vi "SW Arch main.vi"() -> ()   [LabVIEW 2009]
uses:
  <vilib>/Platform/TimedLoop/XDataNode/XDataNode.xnode
  <vilib>/Platform/TimedLoop/XDataNode/nitl_modes.ctl
  <vilib>/Platform/TimedLoop/XDataNode/XDNodeRunTimeDep.lvlib
  <vilib>/Platform/TimedLoop/XDataNode/wakeup.ctl
  <vilib>/Platform/TimedLoop/XDataNode/timing_clust.ctl
  <vilib>/Platform/TimedLoop/XDataNode/loadlvalarms.vi
  <vilib>/rvi/interface/nirviOpenFPGA/nirviOpenFPGA.xnode
  <vilib>/userDefined/High Color/nirio_resource_hc.ctl
  Remote Control/Motor Command.ctl
  TypeDefs/Queue TypeDefs/Motor Instruction.ctl
  TypeDefs/State Machine/Main State.ctl
  <vilib>/LabVIEW Targets/FPGA/cRIO/shared/nicrio_ModuleControls/nicrio_cRIO-9871_DataBitsEnum.ctl
  <vilib>/LabVIEW Targets/FPGA/cRIO/shared/nicrio_ModuleControls/nicrio_cRIO-9871_FlowControlEnum.ctl
  <vilib>/LabVIEW Targets/FPGA/cRIO/shared/nicrio_ModuleControls/nicrio_cRIO-9871_BaudRateEnum.ctl
  <vilib>/LabVIEW Targets/FPGA/cRIO/shared/nicrio_ModuleControls/nicrio_cRIO-9871_ParityEnum.ctl
  <vilib>/LabVIEW Targets/FPGA/cRIO/shared/nicrio_ModuleControls/nicrio_cRIO-9871_StopBitsEnum.ctl
  Remote Control/Message Type.ctl
  FPGA Bitfiles/Q_IGVC_2010.lvproj_FPGA Target_FPGA_MAIN.vi.lvbitx
  TypeDefs/Queue TypeDefs/Motor State.ctl
  <vilib>/FPGAPlugInAG/cRIO-9113/nirviIntfOpen_cRIO-9113.vi
  TypeDefs/Sensor TypeDefs/FPGA Main ref.ctl
  TypeDefs/Sensor TypeDefs/GPS Data.ctl
  TypeDefs/Sensor TypeDefs/SICK Array.ctl
  Remote Control/Control Message.ctl
panel:
  in  "Control Message":T1
  in  "Read Timeout":i32=1000
  in  "Local Port":u16=8800
  out "Run/!RC":bool=TRUE
  out "Main State":T3=enum."Initialize Sensors"
  out "MC VISA resource":refnum<visa-resource-name>="ASRL1::INSTR"
  in  "Motors Init Complete":bool
  out "Motor Queue":refnum<queue>
  in  "RC Command Buffer":T2
  in  "Motors On?":bool
  in  "Sensors Init Complete":bool
  in  "SICK Buffer":T4
  in  "Compass Buffer":dbl=181.1
  in  "Compass Init Complete":bool
  in  "SICK Init Complete":bool
  in  "GPS Init Complete":bool
  in  "GPS Buffer":T5 {"Longitude" format="%#_14g"; "Latitude" format="%#_14g"}
  out "FPGA VI Reference":T6
  in  "Motor Message":string
  out "VFH Queue":refnum<queue>
  out "Communication Queue":refnum<queue>
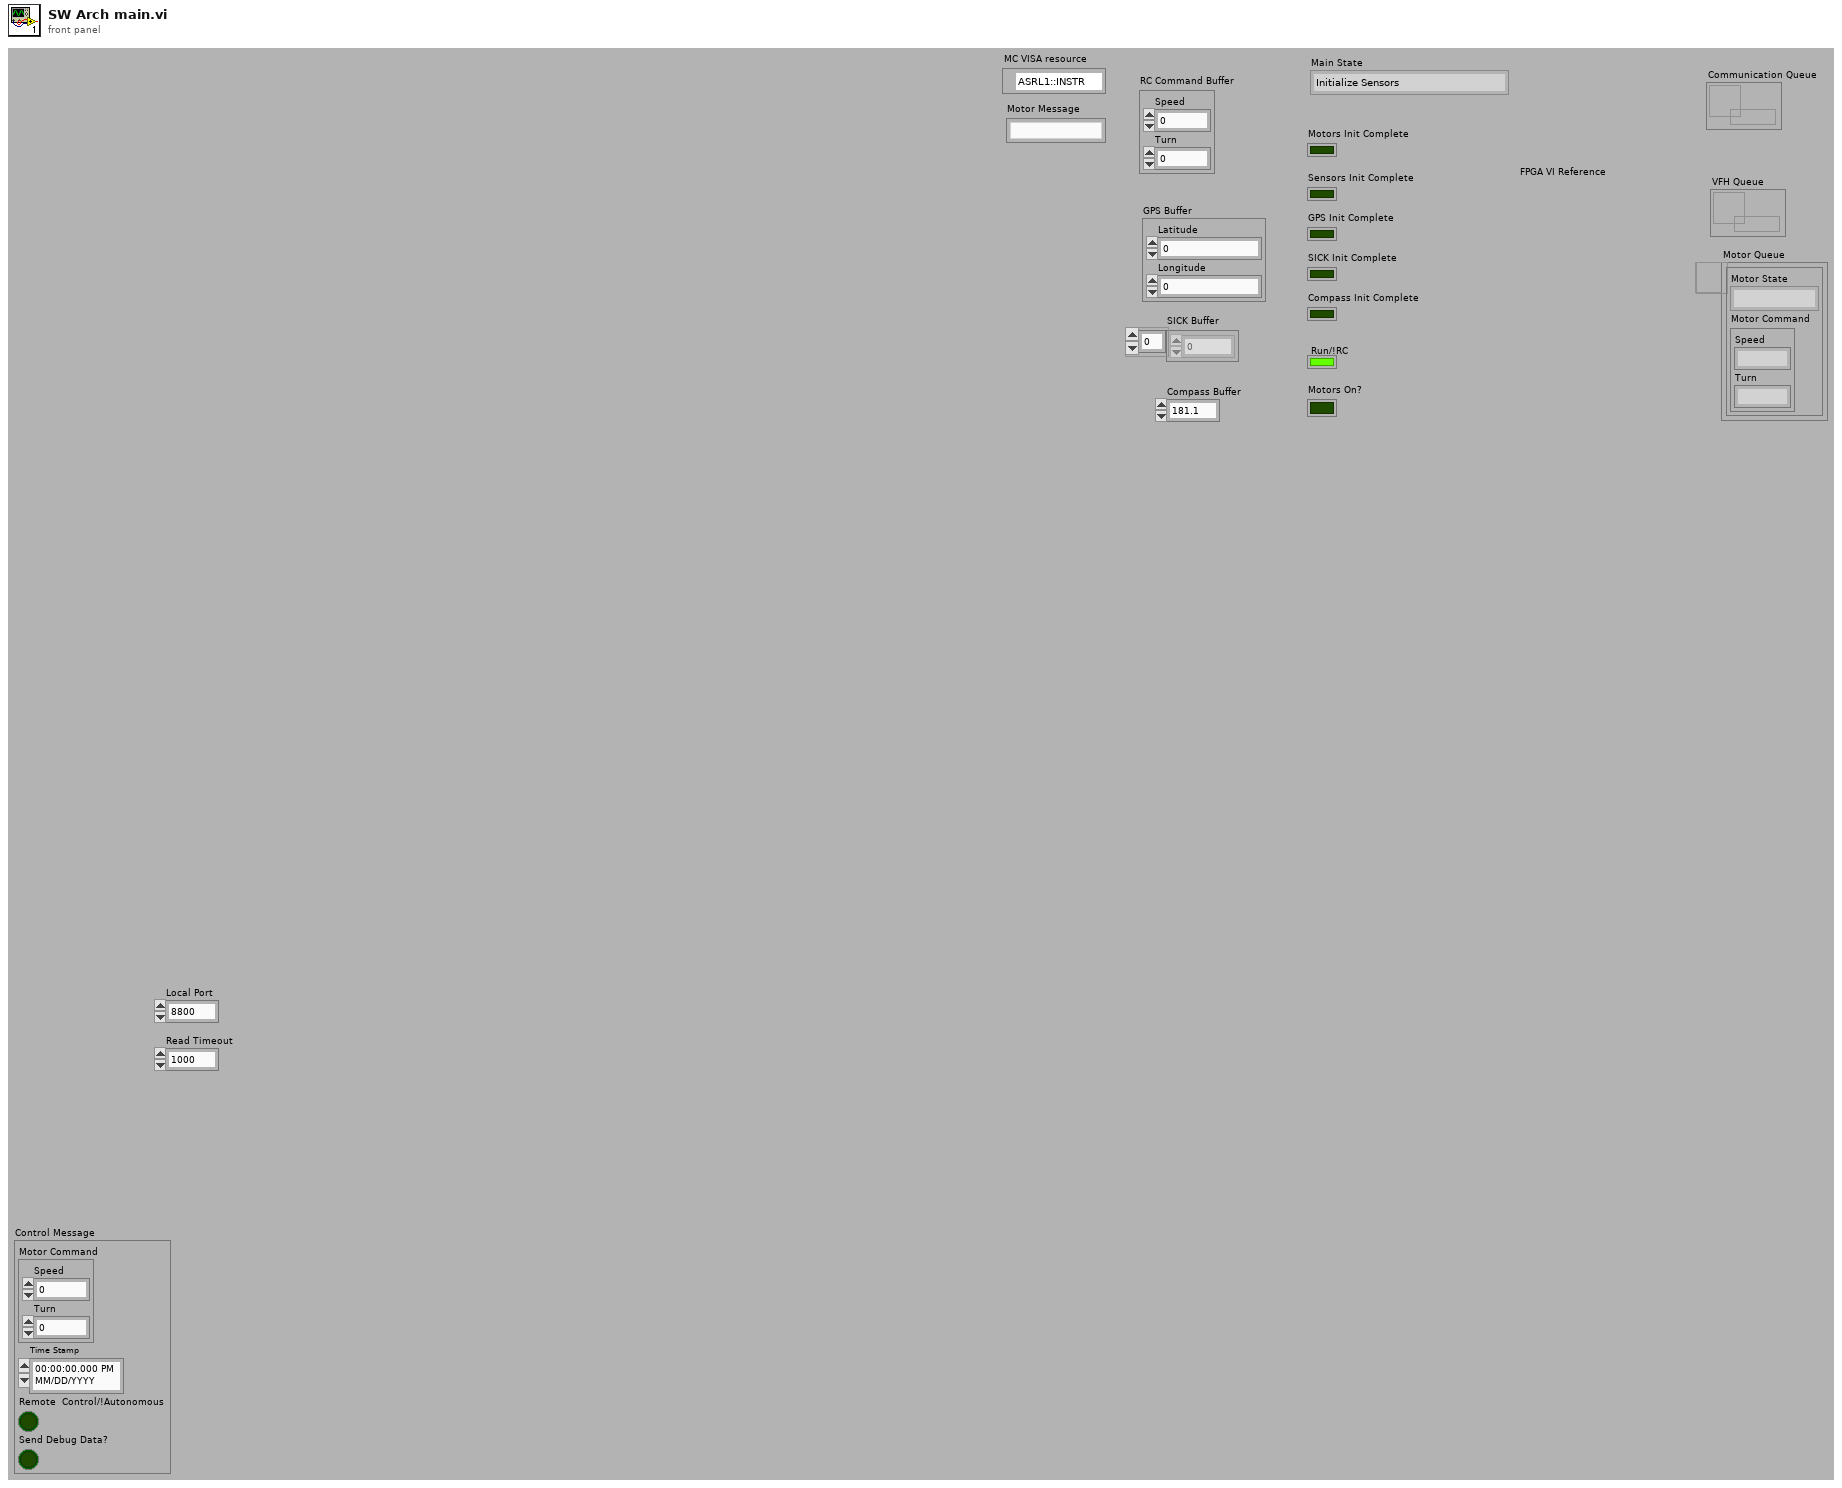
[diagram p1: front panel]
types:
  T1 = typedef "Control Message.ctl" = cluster{"Motor Command":T2, "Time Stamp":timestamp, "Remote  Control/!Autonomous":bool, "Send Debug Data?":bool}
  T2 = typedef "Motor Command.ctl" = cluster{"Speed":i16, "Turn":i16}
  T3 = typedef "Main State.ctl" = enum16{"Wait for Init", "Initialize Sensors", "Wait for Saftey Disable", "Check Saftey", "Wait for GO", "Run", "Remote Control", "Stop"}
  T4 = typedef "SICK Array.ctl" = u16[]
  T5 = typedef "GPS Data.ctl" = cluster{"Latitude":dbl, "Longitude":dbl}
  T6 = typedef "FPGA Main ref.ctl" = refnum<k20>
  T7 = typedef "nicrio_cRIO-9871_StopBitsEnum.ctl" = enum8{"1", "1.5", "2"}
  T8 = typedef "nicrio_cRIO-9871_ParityEnum.ctl" = enum8{"None", "Odd", "Even", "Mark", "Space"}
  T9 = typedef "nicrio_cRIO-9871_BaudRateEnum.ctl" = enum16{"75 bps", "110 bps", "134 bps", "150 bps", "300 bps", "600 bps", "1200 bps", "1800 bps", "2400 bps", "4800 bps", "7200 bps", "9600 bps", "14.4 kbps", "19.2 kbps", "28.8 kbps", "38.4 kbps", "57.6 kbps", "115.2 kbps", "230.4 kbps", "460.8 kbps", "921.6 kbps"}
  T10 = typedef "nicrio_cRIO-9871_FlowControlEnum.ctl" = enum8{"None", "Software (XON / XOFF)", "Hardware (RTS / CTS)"}
  T11 = typedef "nicrio_cRIO-9871_DataBitsEnum.ctl" = enum8{"5", "6", "7", "8"}
  T12 = typedef "nirio_resource_hc.ctl" = tag
  T13 = cluster{"signature":u8[], "vi signatures match":bool, "signature register address":u32, "reset register address":u32, "control register address":u32, "interrupt base address":u32, "Bitstream Version":u32, "DMA Configuration":cluster{"Name":string, "Depth":u32, "Write? (Deprecated:Use Implementation)":bool, "Physical Channel":u32, "Base Address":u32, "Data Width":u32, "Data Type":enum32{"Boolean", "I8", "I16", "I32", "I64", "U8", "U16", "U32", "U64", "FXP"}, "FXP Properties":variant, "Write Window Address":u32, "Implementation":enum16{"niFpgaTargetToHost", "niFpgaHostToTarget", "niFpgaPeerToPeerWriter", "niFpgaPeerToPeerReader", "niCoreTargetToHost", "niCoreHostToTarget"}, "Control Set":u32}[], "run when loaded?":bool, "reset register size in bits":u32, "compilation results xml":string}
  T14 = typedef "Motor Instruction.ctl" = cluster{"Motor State":T15, "Motor Command":T2}
  T15 = typedef "Motor State.ctl" = enum16{"Wait", "Initialize", "Check FET", "Run", "Stop"}
  T16 = typedef "XDNodeRunTimeDep.lvlib/timing_clust.ctl" = cluster{"Expected End [f-1]":u64, "Actual End [f-1]":u64, "Finished Late? [f-1]":bool, "Expected End [i-1]":u64, "Actual End [i-1]":u64, "Finished Late? [i-1]":bool, "Expected Start [i]":u64, "Actual Start [i]":u64, "Expected Start [f]":u64, "Actual Start [f]":u64, "Source Name":string, "Structure Name":string, "Period":i64, "Deadline":i64, "Offset":i64, "Start":i64, "Priority":i32, "Timeout":i32, "Mode":T17, "Wakeup Reason":T18, "Error":errorcluster, "Source Type":string, "Secondary Source Type":string, "Global End Time":u64, "Global Start Time":u64, "Frame Duration":u64, "Iteration Duration":u64, "Assigned CPU":i32, "I/O Scan Engine Mode":u32}
  T17 = typedef "XDNodeRunTimeDep.lvlib/nitl_modes.ctl" = enum32{"No Change", "Process missed periods, maintain original phase", "Discard missed periods, maintain original phase", "Process missed periods, ignore original phase", "Discard missed periods, ignore original phase"}
  T18 = typedef "XDNodeRunTimeDep.lvlib/wakeup.ctl" = enum32{"Normal", "Aborted", "Asynchronous wakeup", "Timing source error", "Timed loop error", "Timeout"}
  T19 = typedef "UDP Base.ctl" = cluster{"UDP Session":refnum<k16>, "UDP Socket Params":T20}
  T20 = typedef "UDP Socket Params.ctl" = cluster{"Local Port":u16, "Read Timeout":i32, "Write Timeout":i32}
  T21 = typedef "Message Type.ctl" = enum16{"Motor Command", "Debug Data"}
  T22 = typedef "UDP Network Location.ctl" = cluster{"IP Address":string, "Port":u16}
  T23 = typedef "Motor Queue.ctl" = cluster{"Motor State":T15, "Motor Command":T2}
  T24 = typedef "EVS GPS Data.ctl" = cluster{"Latitude":dbl, "Longitude":dbl}
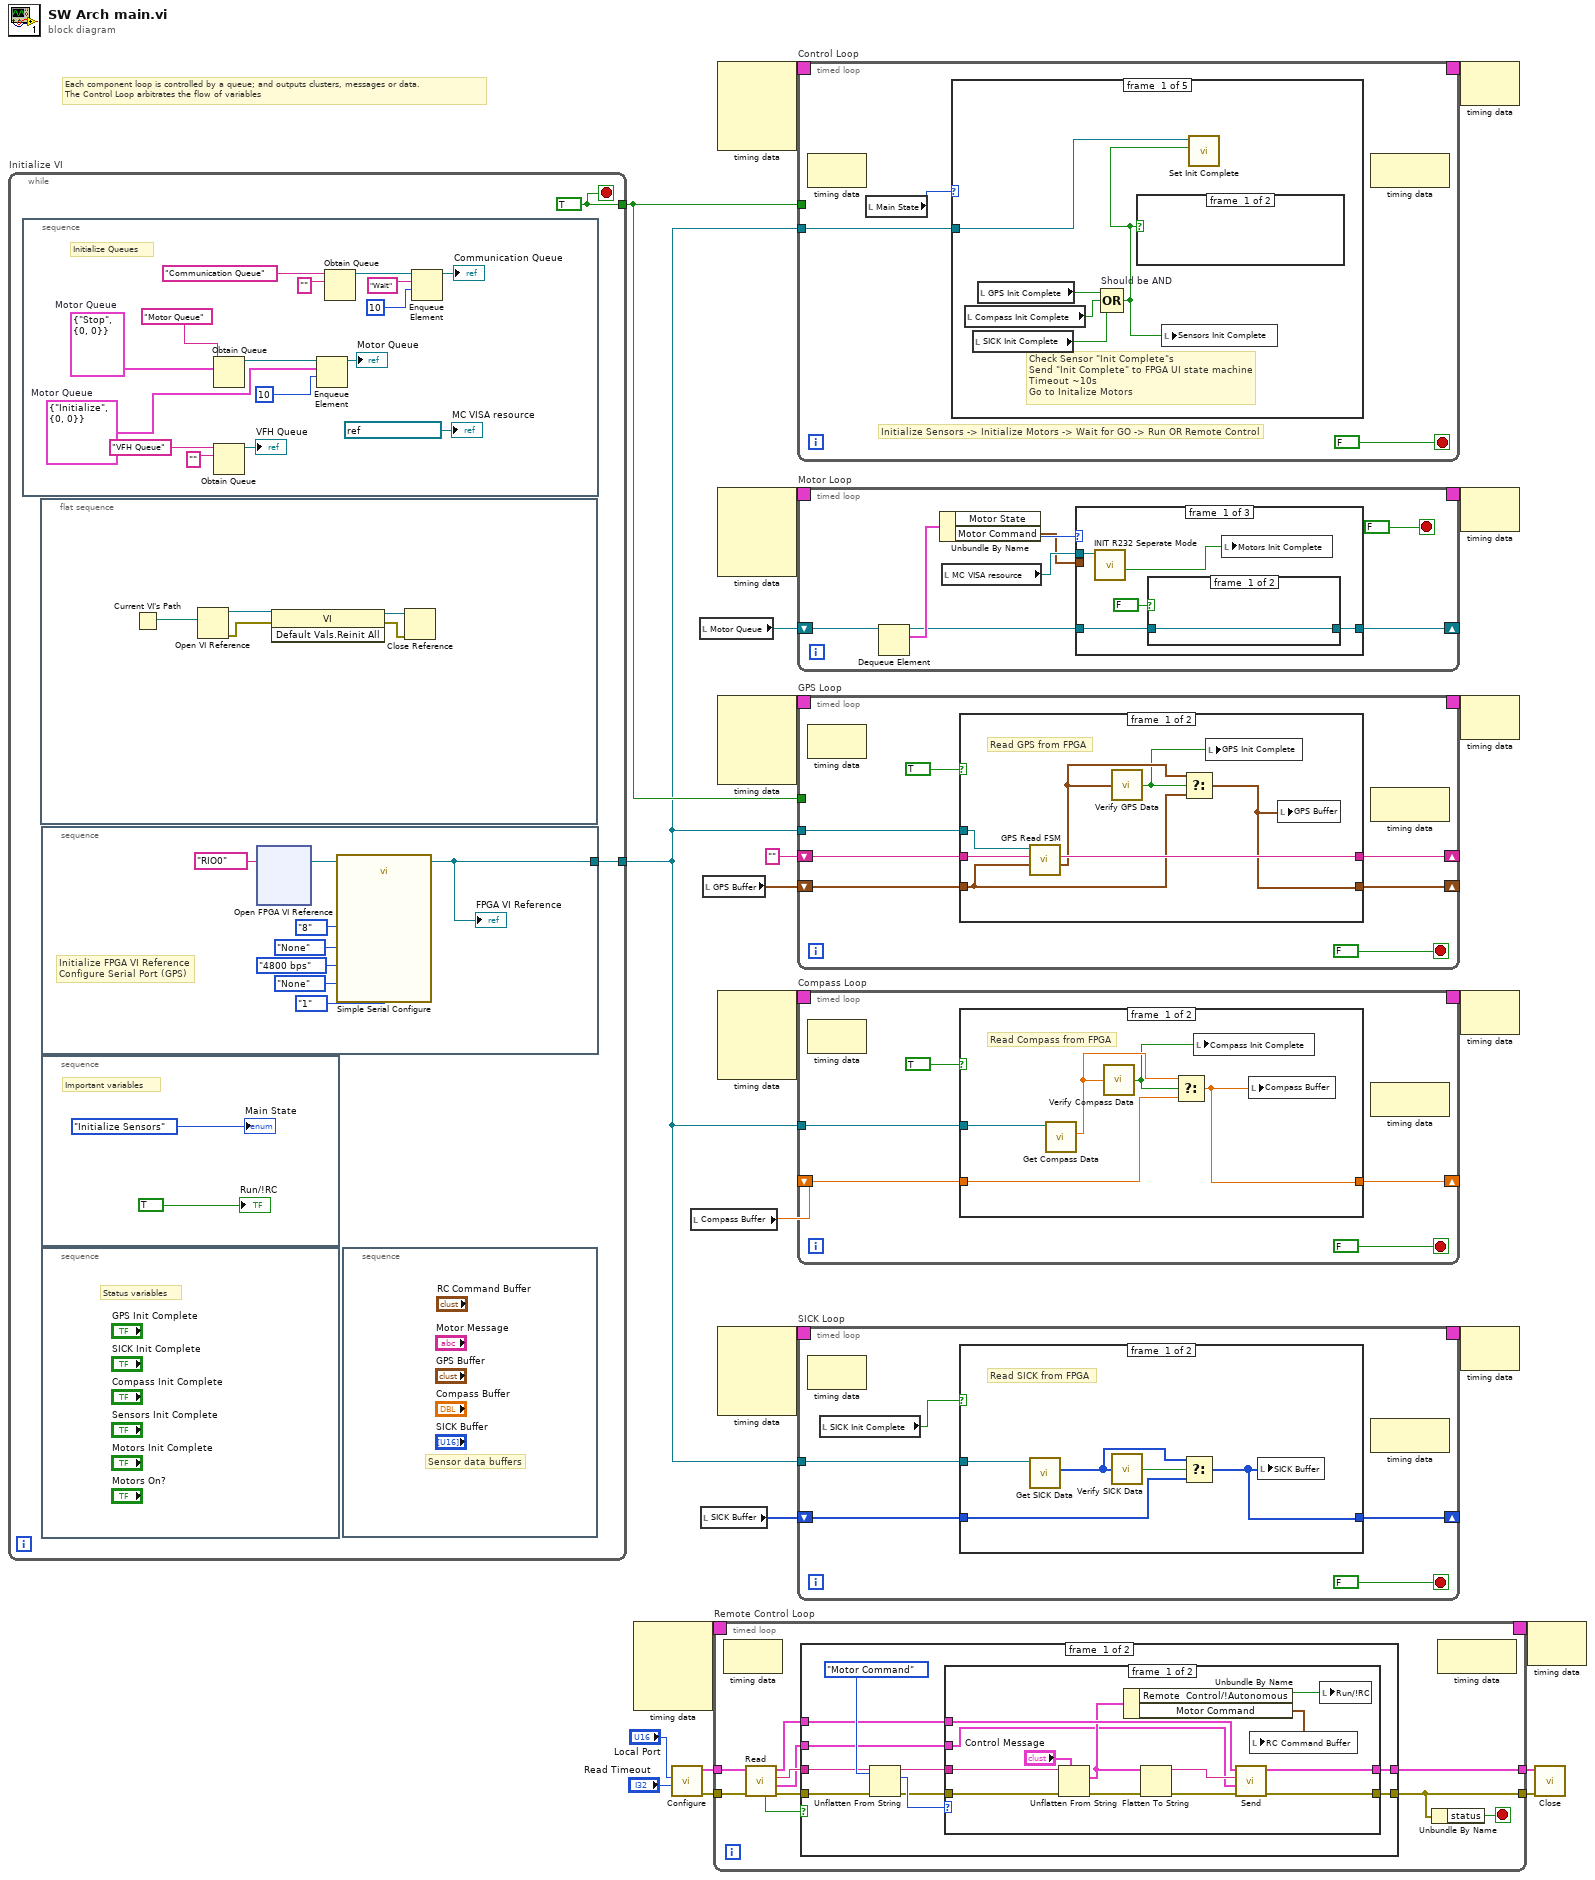
[diagram p0: block diagram]
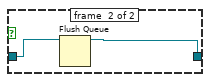
[diagram p4: hidden frame]
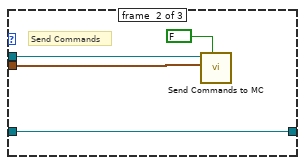
[diagram p5: hidden frame]
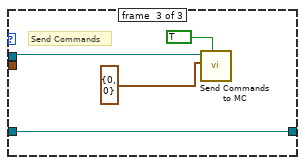
[diagram p6: hidden frame]
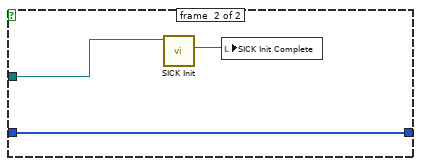
[diagram p7: hidden frame]
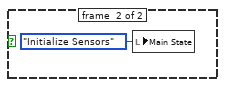
[diagram p10: hidden frame]
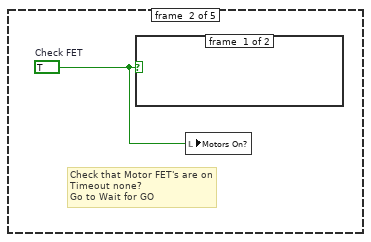
[diagram p11: hidden frame]
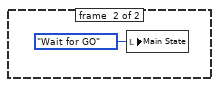
[diagram p12: hidden frame]
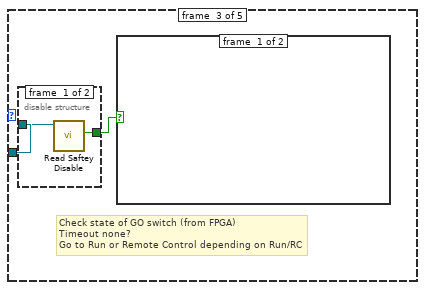
[diagram p13: hidden frame]
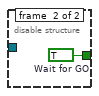
[diagram p14: hidden frame]
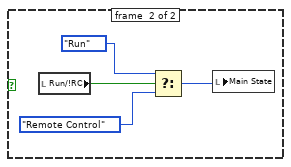
[diagram p15: hidden frame]
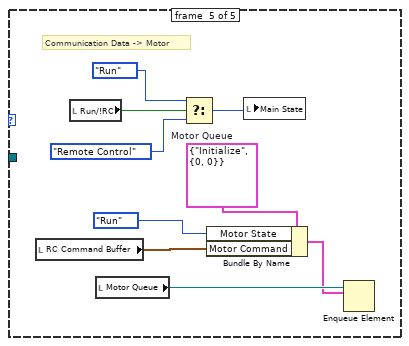
[diagram p17: hidden frame]
diagram:
  # "Each component loop is controlled by a queue; and outputs clusters, messages or data.\nThe Control Loop arbitrates the flow of variables"
  n1 = while "Initialize VI" {
    tunnel: [w27] -> w20
    tunnel: [w26] -> w13
    stop <- w27 stop-if-true
    w27 = TRUE
    n2 = stacked-sequence {
      frame #0 {
        w54 = T14 {"Motor State"=enum."Initialize", "Motor Command"={"Speed"=0, "Turn"=0}}  # Motor Queue
        w57 = T14 {"Motor State"=enum."Stop", "Motor Command"={"Speed"=0, "Turn"=0}}  # Motor Queue
        # "Initialize Queues"
        n3 = Obtain Queue(name (unnamed)="Motor Queue", element data type=w57) -> (queue out=w61:refnum<queue>)  [unwired: 3 in, 2 out]
        n4 = Obtain Queue(name (unnamed)="VFH Queue", element data type="" ("name (unnamed)")) -> (queue out=→"VFH Queue":refnum<queue>)  [unwired: 3 in, 2 out]
        n5 = Enqueue Element(queue=w61, element=w54, timeout in ms (-1)=10) -> (queue out=→"Motor Queue":refnum<queue>)  [unwired: 1 in, 2 out]
        n6 = Obtain Queue(name (unnamed)="Communication Queue", element data type="" ("name (unnamed)")) -> (queue out=w69:refnum<queue>)  [unwired: 3 in, 2 out]
        n7 = Enqueue Element(queue=w69, element="Wait", timeout in ms (-1)=10) -> (queue out=→"Communication Queue":refnum<queue>)  [unwired: 1 in, 2 out]
        "MC VISA resource" <- refnum<visa-resource-name> "ASRL1::INSTR" ("MC VISA resource")
      }
    }
    n8 = flat-sequence {
      frame #0 {
        n9 = Current VI's Path() -> (path=w32:path)
        n10 = Open VI Reference(vi path=w32) -> (vi reference=w30:refnum<vi>, error out=w31:errorcluster)  [unwired: 5 in]
        n11 = invoke class="VI" method="Default Vals.Reinit All"(reference=w30, error in=w31) -> (reference out=w28:refnum<vi>, error out=w29:errorcluster)  [unwired: 1 in, 1 out]
        n12 = Close Reference(reference=w28, error in (no error)=w29) -> ()  [unwired: 1 out]
      }
    }
    n13 = stacked-sequence {
      tunnel: [w40] -> w26
      frame #0 {
        # "Initialize FPGA VI Reference\nConfigure Serial Port (GPS)"
        n14 = xnode "Open FPGA VI Reference"("resource name"=T12 "RIO0") -> ("FPGA VI Reference Out"=w41:refnum<k20>)  [unwired: 1 in, 1 out]
        n15 = call "Simple Serial Configure.vi"("Parity"=nicrio_cRIO-9871_ParityEnum."None", "Stop Bits"=nicrio_cRIO-9871_StopBitsEnum."1", "Flow Control"=nicrio_cRIO-9871_FlowControlEnum."None", "Data Bits"=nicrio_cRIO-9871_DataBitsEnum."8", "Baud Rate"=nicrio_cRIO-9871_BaudRateEnum."4800 bps", "FPGA VI Reference in"=w41) -> ("FPGA VI Reference out"=w40:T6)  [unwired: 4 in, 1 out]
        "FPGA VI Reference" <- w40
      }
    }
    n16 = stacked-sequence {
      frame #0 {
        # "Important variables"
        "Main State" <- Main_State."Initialize Sensors" ("Enum")
        "Run/!RC" <- TRUE ("Run/RC")
      }
    }
    n17 = stacked-sequence {
      frame #0 {
        # "Status variables"
      }
    }
    n18 = stacked-sequence {
      frame #0 {
        # "Sensor data buffers"
      }
    }
  }
  n19 = node-c288() -> (w8:T16)  [unwired: 4 in]
  n20 = call "Configure.vi"("Read Timeout"="Read Timeout", "Local Port"="Local Port") -> ("error out"=w5:errorcluster, "UDP Base out"=w6:T19)  [unwired: 8 in]
  n21 = local read "Compass Buffer"() -> (w16:dbl)
  n22 = local read "Motor Queue"() -> (w9:refnum<queue>)
  n23 = local read "SICK Buffer"() -> (w12:T4)
  n24 = local read "GPS Buffer"() -> (w17:T5)
  n25 = timed-loop "Remote Control Loop" {
    tunnel: w6 -> [w77]
    tunnel: w5 -> [w76]
    tunnel: [w79] -> w3
    tunnel: [w78] -> w4
    timing: w8 -> [_]
    timing-out: [_] -> w7
    stop <- w70 stop-if-true
    n26 = node-c288() -> ()  [unwired: 1 in, 1 out]
    n27 = call "Read.vi"("error in (no error)"=w76, "UDP Base in"=w77) -> ("error out"=w74:errorcluster, "Network Location"=w71:T22, "Receive Data"=w73:string, "UDP Base out"=w75:T19, "Timeout"=w72:bool)  [unwired: 4 in, 1 out]
    n28 = case shown="False" w72 {
      tunnel: [w89 w107] -> w79
      tunnel: [w88 w108] -> w78
      tunnel: w75 -> [w85 w108]
      tunnel: w74 -> [w84 w107]
      tunnel: w73 -> [w83 _]
      tunnel: w71 -> [w82 _]
      frame #0 {
        n29 = Unflatten From String(type=Message_Type."Motor Command" ("Message Type"), binary string=w83, error in (no error)=w84) -> (rest of the binary string=w86:string, value=w90:T21, error out=w87:errorcluster)  [unwired: 2 in]
        n30 = case shown="\"Motor Command\", Default" w90 {
          tunnel: [w98 w106] -> w89
          tunnel: [w99 w105] -> w88
          tunnel: w87 -> [w104 w106]
          tunnel: w86 -> [w103 _]
          tunnel: w85 -> [w96 w105]
          tunnel: w82 -> [w94 _]
          frame #0 {
            n31 = Unflatten From String(type="Control Message", binary string=w103, error in (no error)=w104) -> (value=w95:T1, error out=w102:errorcluster)  [unwired: 2 in, 1 out]
            n32 = Unbundle By Name(w95) -> ("Remote  Control/!Autonomous"=w92:bool, "Motor Command"=w93:T2)
            n33 = Flatten To String(anything=w95, error in (no error)=w102) -> (data string=w97:string, error out=w100:errorcluster)  [unwired: 2 in, 1 out]
            n34 = call "Send.vi"("error in (no error)"=w100, "Destination Location"=w94, "Send Data"=w97, "UDP Base in"=w96) -> ("error out"=w98:errorcluster, "UDP Base out"=w99:T19)  [unwired: 5 in, 1 out]
            n35 = local write "RC Command Buffer"(w93) -> ()
            n36 = local write "Run/!RC"(w92) -> ()
          }
          frame #1 {
          }
        }
      }
      frame #1 {
      }
    }
    n37 = Unbundle By Name(w79) -> ("status"=w70:bool)
    n38 = node-c288() -> ()  [unwired: 1 in, 1 out]
  }
  n39 = node-c288() -> (w25:T16)  [unwired: 4 in]
  n40 = node-c288() -> (w11:T16)  [unwired: 4 in]
  n41 = node-c288() -> (w23:T16)  [unwired: 4 in]
  n42 = node-c288() -> (w19:T16)  [unwired: 4 in]
  n43 = node-c288() -> (w15:T16)  [unwired: 4 in]
  n44 = timed-loop "Control Loop" {
    tunnel: w20 -> [_]
    timing: w25 -> [_]
    timing-out: [_] -> w24
    tunnel: w13 -> [w109]
    stop <- FALSE stop-if-true
    # "Initialize Sensors -> Initialize Motors -> Wait for GO -> Run OR Remote Control"
    n45 = node-c288() -> ()  [unwired: 1 in, 1 out]
    n46 = local read "Main State"() -> (w110:T3)
    n47 = case shown="\"Wait for GO\"" w110 {
      tunnel: w109 -> [w118 _ w123 _ _]
      frame #0 {
        # "Check Sensor \"Init Complete\"s\nSend \"Init Complete\" to FPGA UI state machine\nTimeout ~10s\nGo to Initalize Motors"
        n48 = local read "Compass Init Complete"() -> (w115:bool)
        n49 = local read "SICK Init Complete"() -> (w116:bool)
        n50 = local read "GPS Init Complete"() -> (w117:bool)
        n51 = Compound Arithmetic op=OR "Should be AND"(w117, w115, w116) -> (w114:bool)
        n52 = case shown="True" w114 {
          frame #0 {
          }
          frame #1 {
            n53 = local write "Main State"(Main_State."Initialize Sensors" ("Main State")) -> ()
          }
        }
        n54 = local write "Sensors Init Complete"(w114) -> ()
        n55 = call "Set Init Complete.vi"("Initialization Complete"=w114, "FPGA VI Reference in"=w118) -> ()  [unwired: 8 in, 2 out]
      }
      frame #1 {
        w120 = TRUE  # Check FET
        # "Check that Motor FET's are on\nTimeout none?\nGo to Wait for GO"
        n56 = case shown="True" w120 {
          frame #0 {
          }
          frame #1 {
            n57 = local write "Main State"(Main_State."Wait for GO" ("Main State")) -> ()
          }
        }
        n58 = local write "Motors On?"(w120) -> ()
      }
      frame #2 {
        # "Check state of GO switch (from FPGA)\nTimeout none?\nGo to Run or Remote Control depending on Run/RC"
        n59 = disable-structure shown="Enabled" {
          disable-tunnel: w123 -> [w125 _]
          disable-tunnel: [w124 w126] -> w122
          frame #0 {
            n60 = call "Read Saftey Disable.vi"("FPGA VI Reference in"=w125) -> ("GO"=w124:bool)  [unwired: 7 in, 2 out]
          }
          frame #1 {
            w126 = TRUE  # Wait for GO
          }
        }
        n61 = case shown="True" w122 {
          frame #0 {
          }
          frame #1 {
            n62 = local read "Run/!RC"() -> (w130:bool)
            n63 = Select(t=Main_State."Run" ("Main State"), s=w130, f=Main_State."Remote Control" ("Main State")) -> (s? t:f=w129:T3)
            n64 = local write "Main State"(w129) -> ()
          }
        }
      }
      frame #3 {
        # "Run Sensor\nRun VFH on new imge data\nSensor Data -> VFH\nVFH Data -> Motor"
      }
      frame #4 {
        w137 = T14 {"Motor State"=enum."Initialize", "Motor Command"={"Speed"=0, "Turn"=0}}  # Motor Queue
        # "Communication Data -> Motor"
        n65 = local read "RC Command Buffer"() -> (w138:T2)
        n66 = local read "Run/!RC"() -> (w134:bool)
        n67 = local read "Motor Queue"() -> (w139:refnum<queue>)
        n68 = Select(t=Main_State."Run" ("Main State"), s=w134, f=Main_State."Remote Control" ("Main State")) -> (s? t:f=w133:T3)
        n69 = Bundle By Name(cluster=w137, "Motor State"=enum16{"Initialize", "Run", "Stop"}."Run", "Motor Command"=w138) -> (w135:T14)
        n70 = local write "Main State"(w133) -> ()
        n71 = Enqueue Element(queue=w139, element=w135) -> ()  [unwired: 2 in, 3 out]
      }
    }
    n72 = node-c288() -> ()  [unwired: 1 in, 1 out]
  }
  n73 = timed-loop "Motor Loop" {
    timing: w11 -> [_]
    timing-out: [_] -> w10
    shift-right: [w141] -> _
    shift-left: w9 -> [w143]
    stop <- FALSE stop-if-true
    n74 = Dequeue Element(queue=w143) -> (queue out=w142:refnum<queue>, element=w146:T23)  [unwired: 2 in, 2 out]
    n75 = Unbundle By Name(w146) -> ("Motor State"=w145:T15, "Motor Command"=w140:T2)
    n76 = local read "MC VISA resource"() -> (w144:refnum<visa-resource-name>)
    n77 = case shown="\"Run\"" w145 {
      tunnel: w144 -> [w152 w158 w162]
      tunnel: w142 -> [w150 w159 w163]
      tunnel: [w149 w159 w163] -> w141
      tunnel: w140 -> [_ w156 _]
      frame #0 {
        n78 = call "INIT R232 Seperate Mode.vi"("MC VISA resource in"=w152) -> ("MC Init Complete"=w151:bool)  [unwired: 8 in, 2 out]
        n79 = case shown="False" FALSE {
          tunnel: w150 -> [w153 w155]
          tunnel: [w153 w154] -> w149
          frame #0 {
          }
          frame #1 {
            n80 = Flush Queue(queue=w155) -> (queue out=w154:refnum<queue>)  [unwired: 1 in, 2 out]
          }
        }
        n81 = local write "Motors Init Complete"(w151) -> ()
      }
      frame #1 {
        # "Send Commands"
        n82 = call "Send Commands to MC.vi"("Pause Motors"=FALSE, "Motor Command"=w156, "MC refrence in"=w158) -> ()  [unwired: 4 in, 2 out]
      }
      frame #2 {
        # "Send Commands"
        n83 = call "Send Commands to MC.vi"("Pause Motors"=TRUE, "Motor Command"=T2 {"Speed"=0, "Turn"=0}, "MC refrence in"=w162) -> ()  [unwired: 4 in, 2 out]
      }
    }
  }
  n84 = timed-loop "GPS Loop" {
    timing: w23 -> [_]
    timing-out: [_] -> w22
    shift-right: [w166] -> _
    shift-left: "" ("header buffer") -> [w170]
    tunnel: w13 -> [w169]
    shift-right: [w167] -> _
    shift-left: w17 -> [w168]
    tunnel: w20 -> [_]
    stop <- FALSE stop-if-true
    n85 = node-c288() -> ()  [unwired: 1 in, 1 out]
    n86 = case shown="True" TRUE {
      tunnel: w170 -> [w181 w182]
      tunnel: w169 -> [w180 _]
      tunnel: w168 -> [w177 w183]
      tunnel: [w176 w183] -> w167
      tunnel: [w179 w182] -> w166
      frame #0 {
        # "Read GPS from FPGA"
        n87 = call "GPS Read FSM.vi"("GPS Buffer in"=w177, "header buffer in"=w181, "FPGA VI Reference in"=w180) -> ("GPS Buffer out"=w178:T24, "header buffer out"=w179:string)  [unwired: 4 in, 3 out]
        n88 = call "Verify GPS Data.vi"("GPS Point"=w178) -> ("Data OK?"=w175:bool)
        n89 = Select(t=w178, s=w175, f=w177) -> (s? t:f=w176:T5)
        n90 = local write "GPS Init Complete"(w175) -> ()
        n91 = local write "GPS Buffer"(w176) -> ()
      }
      frame #1 {
      }
    }
    n92 = node-c288() -> ()  [unwired: 1 in, 1 out]
  }
  n93 = timed-loop "Compass Loop" {
    timing: w19 -> [_]
    timing-out: [_] -> w18
    tunnel: w13 -> [w186]
    shift-right: [w184] -> _
    shift-left: w16 -> [w185]
    stop <- FALSE stop-if-true
    n94 = node-c288() -> ()  [unwired: 1 in, 1 out]
    n95 = case shown="True" TRUE {
      tunnel: w186 -> [w195 _]
      tunnel: w185 -> [w193 w196]
      tunnel: [w191 w196] -> w184
      frame #0 {
        # "Read Compass from FPGA"
        n96 = call "Get Compass Data.vi"("FPGA_MAIN ref in"=w195) -> ("Compass Bearing"=w194:dbl)  [unwired: 8 in, 2 out]
        n97 = call "Verify Compass Data.vi"("Compass Data"=w194) -> ("Data OK?"=w192:bool)
        n98 = Select(t=w194, s=w192, f=w193) -> (s? t:f=w191:dbl)
        n99 = local write "Compass Init Complete"(w192) -> ()
        n100 = local write "Compass Buffer"(w191) -> ()
      }
      frame #1 {
      }
    }
    n101 = node-c288() -> ()  [unwired: 1 in, 1 out]
  }
  n102 = timed-loop "SICK Loop" {
    timing: w15 -> [_]
    timing-out: [_] -> w14
    tunnel: w13 -> [w200]
    shift-right: [w198] -> _
    shift-left: w12 -> [w199]
    stop <- FALSE stop-if-true
    n103 = node-c288() -> ()  [unwired: 1 in, 1 out]
    n104 = local read "SICK Init Complete"() -> (w197:bool)
    n105 = case shown="False" w197 {
      tunnel: w200 -> [w208 w210]
      tunnel: w199 -> [w205 w211]
      tunnel: [w204 w211] -> w198
      frame #0 {
        # "Read SICK from FPGA"
        n106 = call "Get SICK Data.vi"("FPGA_MAIN ref in"=w208) -> ("SICK Data"=w206:T4)  [unwired: 7 in, 3 out]
        n107 = call "Verify SICK Data.vi"("SICK Data"=w206) -> ("Data OK?"=w207:bool)
        n108 = Select(t=w206, s=w207, f=w205) -> (s? t:f=w204:T4)
        n109 = local write "SICK Buffer"(w204) -> ()
      }
      frame #1 {
        n110 = call "SICK Init.vi"("FPGA_MAIN ref in"=w210) -> ("Init Success"=w209:bool)  [unwired: 8 in, 2 out]
        n111 = local write "SICK Init Complete"(w209) -> ()
      }
    }
    n112 = node-c288() -> ()  [unwired: 1 in, 1 out]
  }
  n113 = node-c288(w24) -> ()  [unwired: 1 out]
  n114 = node-c288(w10) -> ()  [unwired: 1 out]
  n115 = node-c288(w22) -> ()  [unwired: 1 out]
  n116 = node-c288(w18) -> ()  [unwired: 1 out]
  n117 = node-c288(w14) -> ()  [unwired: 1 out]
  n118 = node-c288(w7) -> ()  [unwired: 1 out]
  n119 = call "Close.vi"("error in (no error)"=w3, "Cluster of class private data"=w4) -> ()  [unwired: 9 in, 1 out]
